vi "ConvertItemListToTraceFormatElements.vi"(11 "Item List":string) -> (3 "Trace Format Elements":T1[](array[typedef]))   [LabVIEW 8.6, in "Keithley-6482-Visa.lvlib"]
uses:
  Keithley-6482-Visa.lvlib
  Public/Controls/TraceFormatElement.ctl
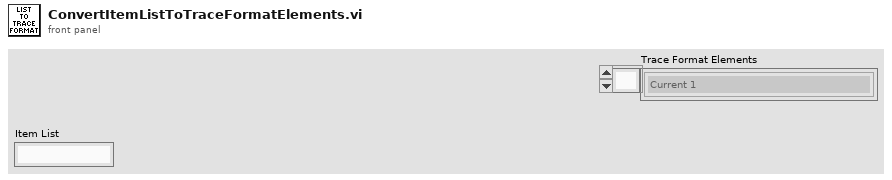
[diagram p1: front panel]
types:
  T1 = typedef "Keithley-6482-Visa.lvlib/TraceFormatElement.ctl" = enum16{"Current 1", "Current 2", "Calculate 1", "Calculate 2", "Calculate 3", "Calculate 4", "Calculate 5", "Calculate 6", "Calculate 7", "Time", "Status", "All", "Default"}
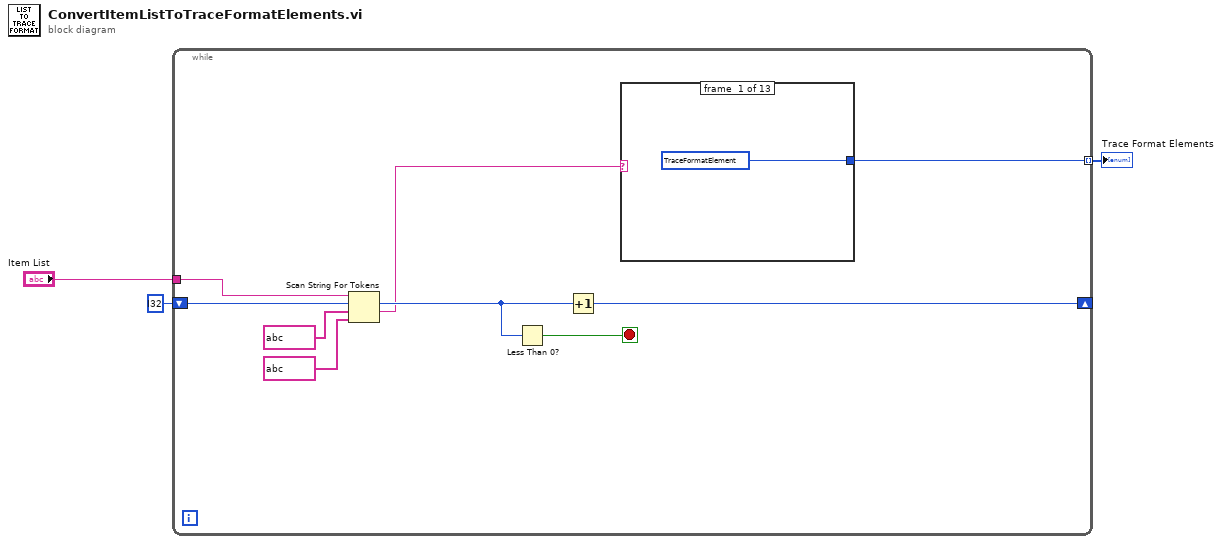
[diagram p0: block diagram]
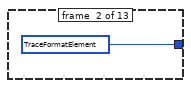
[diagram p2: hidden frame]
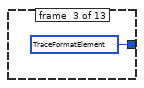
[diagram p3: hidden frame]
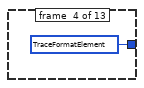
[diagram p4: hidden frame]
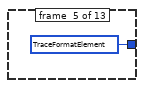
[diagram p5: hidden frame]
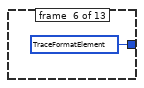
[diagram p6: hidden frame]
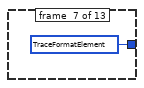
[diagram p7: hidden frame]
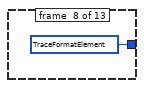
[diagram p8: hidden frame]
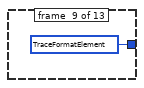
[diagram p9: hidden frame]
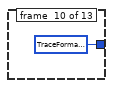
[diagram p10: hidden frame]
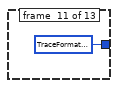
[diagram p11: hidden frame]
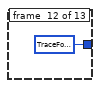
[diagram p12: hidden frame]
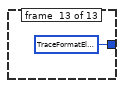
[diagram p13: hidden frame]
diagram:
  n1 = while {
    shift-right: [w6] -> _
    shift-left: i32 ? ("offset past token") -> [w12]
    tunnel: "Item List" -> [w9]
    tunnel: [w4] -> w1 mode=indexing
    stop <- w8 stop-if-true
    n2 = Scan String For Tokens(6:string[] ? ("delimiters (\\s,\\t,\\r,\\n)"), 7:string[] ? ("delimiters (\\s,\\t,\\r,\\n)"), 8:w12, 9:w9) -> (1:w5:string, 2:w7:i32)  [unwired: 2 in, 2 out]
    n3 = Less Than 0?(x=w7) -> (x < 0?=w8:bool)
    n4 = Increment(x=w7) -> (x+1=w6:i32)
    n5 = case shown="\"DEF\"" w5 {
      tunnel: [T1 ? ("Trace Format Element") T1 ? ("Trace Format Element") T1 ? ("Trace Format Element") T1 ? ("Trace Format Element") T1 ? ("Trace Format Element") T1 ? ("Trace Format Element") T1 ? ("Trace Format Element") T1 ? ("Trace Format Element") T1 ? ("Trace Format Element") T1 ? ("Trace Format Element") T1 ? ("Trace Format Element") T1 ? ("Trace Format Element") T1 ? ("Trace Format Element")] -> w4
      frame #0 {
      }
      frame #1 {
      }
      frame #2 {
      }
      frame #3 {
      }
      frame #4 {
      }
      frame #5 {
      }
      frame #6 {
      }
      frame #7 {
      }
      frame #8 {
      }
      frame #9 {
      }
      frame #10 {
      }
      frame #11 {
      }
      frame #12 {
      }
    }
  }
  "Trace Format Elements" <- w1
